vi "sonar222.vi"() -> ()   [LabVIEW 2020]
doc: "Use this template to build a producer/consumer design pattern. Use this template when you need to execute a process, such as data analysis, when a data source, such as a triggered acquisition, produces data at an uneven rate and you need to execute the process when the data becomes available."
uses:
  <vilib>/picture/picture.llb/imagedata.ctl
  <vilib>/MakerHub/LINX/Public/Utilities/Open Serial.vi
  <vilib>/MakerHub/LINX/Public/Sensors/Motion/Servo/Servo Open One Channel.vi
  <vilib>/MakerHub/LINX/Public/Sensors/Motion/Servo/Servo Set Pulse Width One Channel.vi
  <vilib>/MakerHub/LINX/Public/Sensors/Motion/Servo/Servo Close One Channel.vi
  <vilib>/MakerHub/LINX/LMH-LINX.lvlib
  <vilib>/MakerHub/LINX/Public/Sensors/Motion/Servo/Servo.lvlib
  <vilib>/MakerHub/LINX/Public/Sensors/Distance/Ultrasonic/Ultrasonic.lvlib
panel:
  out "2D picture":picture
  in  "STOP":bool
  out "Distance":dbl
  in  "Echo Pin":u8
  in  "Trig Pin":u8
  in  "Servo Pin":i32=10
  out "Angle":dbl
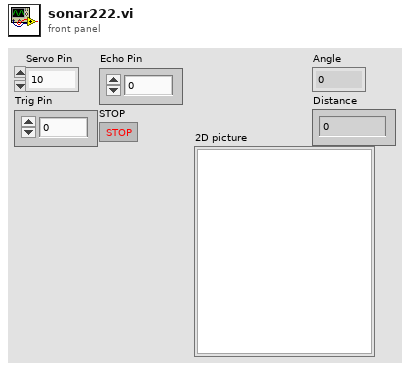
[diagram p1: front panel]
types:
  T1 = typedef "imagedata.ctl" = cluster{"image type":i32, "image depth":i32, "image":u8[], "mask":u8[], "colors":u32[], "Rectangle":cluster{"left":i16, "top":i16, "right":i16, "bottom":i16}}
  T2 = typedef "LMH-LINX.lvlib/LINX Ref.ctl" = cluster{"IO":T3, "Interface":T4, "LINX Device Config":T5}
  T3 = typedef "LMH-LINX.lvlib/Platform.ctl" = enum16{"Remote", "Local"}
  T4 = typedef "LMH-LINX.lvlib/Interface.ctl" = enum16{"Serial", "TCP"}
  T5 = typedef "LMH-LINX.lvlib/Device.lvlib/LINX Device Config.ctl" = cluster{"Interface":T4, "COM Port":refnum<visa-resource-name>, "TCP Configuration":T6, "Device Family":u8, "Device ID":u8, "Device Name":string, "TCP Ref":refnum<k5>, "Channels":T7}
  T6 = typedef "LMH-LINX.lvlib/Device.lvlib/TCP Config.ctl" = cluster{"IP Address":string, "Port":u16}
  T7 = typedef "LMH-LINX.lvlib/Channels.ctl" = cluster{"DI":u8[], "DO":u8[], "AI":u8[], "AO":u8[], "PWM":u8[], "QE":u8[], "UART":u8[], "I2C 2":u8[], "SPI":u8[], "CAN":u8[], "Servo":u8[], "AI Ref (V)":dbl, "AI Resolution (Bits)":u8, "AO Ref (V)":dbl, "AO Resolution (Bits)":u8}
  T8 = cluster{"maximum":dbl, "minimum":dbl, "clip to min":bool, "log?(F)":bool, "grid color":u32, "plot color":u32, "format and precision":cluster{"format":enum8{"Decimal", "Scientific", "Engineering", "Binary", "Octal", "Hex"}, "precision":u8}, "visible section":u16}
  T9 = typedef "LVBoundsTypeDef.ctl" = cluster{"Width":u32, "Height":u32}
  T10 = cluster{"pixel center":cluster{"x":i16, "y":i16}, "scale factors":cluster{"a":dbl, "b":dbl, "log?":bool}, "grid color":u32, "start angle":dbl, "end angle":dbl, "tick length":i16, "pixel radius":i32}
  T11 = cluster{"Distance (cm)":dbl, "Angle (deg)":dbl}[]
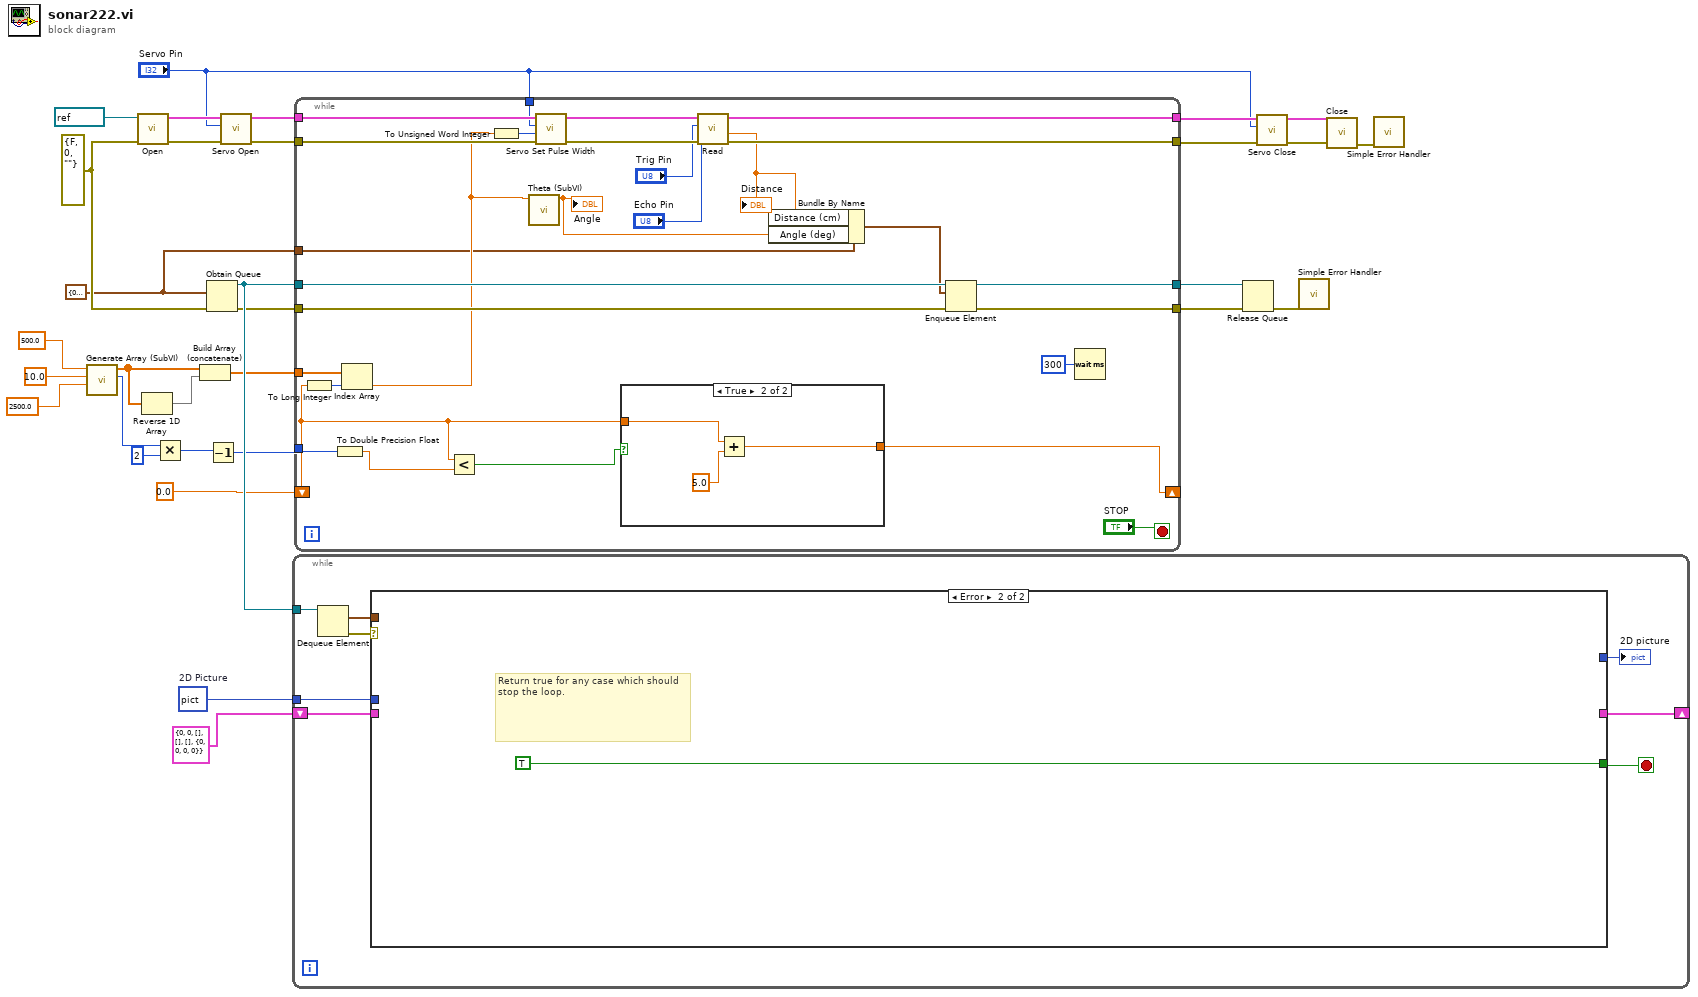
[diagram p0: block diagram]
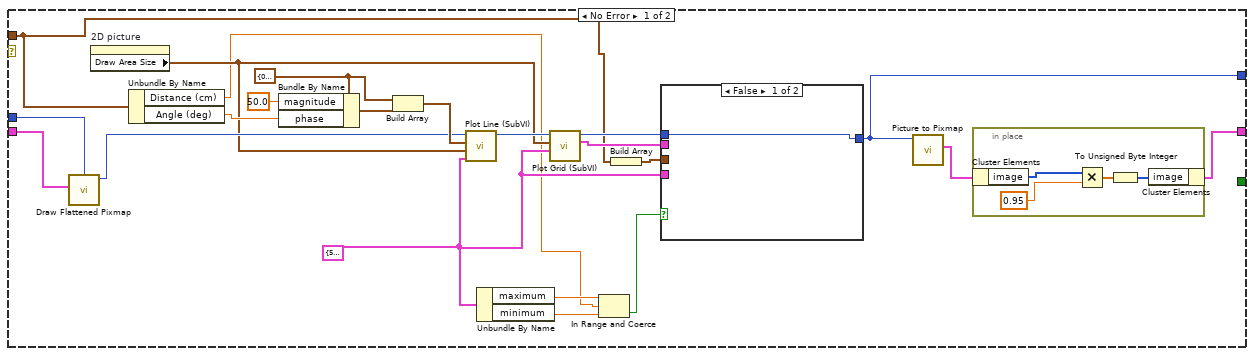
[diagram p2: hidden frame]
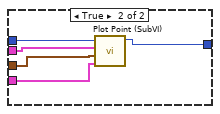
[diagram p3: hidden frame]
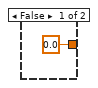
[diagram p4: hidden frame]
diagram:
  w1 = picture data[5B]  # 2D Picture
  w3 = cluster{"Distance (cm)":dbl, "Angle (deg)":dbl} {"Distance (cm)"=0.0, "Angle (deg)"=0.0}
  w17 = errorcluster {"status"=FALSE, "code"=0, "source"=""} ("Error Cluster In")
  n1 = call "Generate Array (SubVI).vi"("Final"=2500.0, "Step"=10.0, "Initial"=500.0) -> ("Array size"=w7:i32, "Array out"=w10:dbl[])  [unwired: 6 in, 1 out]
  n2 = call-poly <vilib>:"Open.vi"("Error In"=w17, "Serial Port"=refnum<visa-resource-name> "N/A") -> ("Error Out"=w23:errorcluster, "LINX Resource"=w27:T2)  [unwired: 7 in, 1 out]
  n3 = Reverse 1D Array(array=w10) -> (reversed array=w11:dbl[])
  n4 = Multiply(x=w7, y=2) -> (x*y=w5:i32)
  n5 = Build Array (concatenate)(w10, w11) -> (w9:dbl[])
  n6 = Obtain Queue(element data type=w3, error in (no error)=w17) -> (queue out=w31:refnum<queue>, error out=w30:errorcluster)  [unwired: 3 in, 1 out]
  n7 = Decrement(x=w5) -> (x-1=w4:i32)
  n8 = call-poly <vilib>:"Servo Open.vi"("Error In"=w23, "Servo Channel"="Servo Pin", "LINX Resource"=w27) -> ("Error Out"=w22:errorcluster, "LINX Resource"=w26:T2)  [unwired: 7 in]
  n9 = while {
    tunnel: w31 -> [w39]
    tunnel: w1 -> [w35]
    shift-right: [w33] -> _
    shift-left: T1 {"image type"=0, "image depth"=0, "image"=[], "mask"=[], "colors"=[], "Rectangle"={"left"=0, "top"=0, "right"=0, "bottom"=0}} -> [w36]
    stop <- w34 stop-if-true
    n10 = Dequeue Element(queue=w39) -> (element=w37:cluster{"Distance (cm)":dbl, "Angle (deg)":dbl}, error out=w38:errorcluster)  [unwired: 2 in, 2 out]
    n11 = case shown="Error" w38 {
      tunnel: w37 -> [w48 _]
      tunnel: [_ TRUE] -> w34
      tunnel: w36 -> [w61 _]
      tunnel: w35 -> [w55 _]
      tunnel: [w46 _] -> w33
      tunnel: [w45 _] -> w32
      frame No Error {
        w44 = T8 {"maximum"=50.0, "minimum"=0.0, "clip to min"=TRUE, "log?(F)"=FALSE, "grid color"=9868950, "plot color"=65280, "format and precision"={"format"=enum."Decimal", "precision"=0}, "visible section"=4} ("Polar Graph Attributes")
        w58 = cluster{"magnitude":dbl, "phase":dbl} {"magnitude"=0.0, "phase"=0.0}
        n12 = call <vilib>:"Draw Flattened Pixmap.vi"("image data"=w61, "picture"=w55) -> ("new picture"=w54:picture)  [unwired: 7 in]
        n13 = property on="2D picture" class="Pict"() -> ("Draw Area Size"=w52:T9)  [unwired: 2 in, 2 out]
        n14 = Unbundle By Name(w48) -> ("Distance (cm)"=w41:dbl, "Angle (deg)"=w60:dbl)
        n15 = Bundle By Name(cluster=w58, "magnitude"=50.0, "phase"=w60) -> (w57:cluster{"magnitude":dbl, "phase":dbl})
        n16 = Build Array(w58, w57) -> (w56:cluster{"magnitude":dbl, "phase":dbl}[])
        n17 = call "Plot Line (SubVI).vi"("Polar Graph Attributes"=w44, "Draw Area Size"=w52, "Polar Array"=w56, "new picture in"=w54) -> ("new picture out"=w53:picture)  [unwired: 7 in]
        n18 = Unbundle By Name(w44) -> ("maximum"=w43:dbl, "minimum"=w42:dbl)
        n19 = call "Plot Grid (SubVI).vi"("Polar Graph Attributes"=w44, "Draw Area Size"=w52, "new picture in"=w53) -> ("grid measurements"=w50:T10, "new picture out"=w51:picture)  [unwired: 7 in]
        n20 = In Range and Coerce(upper limit=w43, x=w41, lower limit=w42) -> (In Range?=w40:bool)  [unwired: 1 out]
        n21 = Build Array(w48) -> (w49:T11)
        n22 = case shown="False" w40 {
          tunnel: w51 -> [w66 w71]
          tunnel: w50 -> [_ w70]
          tunnel: w49 -> [_ w69]
          tunnel: w44 -> [_ w68]
          tunnel: [w66 w67] -> w45
          frame False {
          }
          frame True {
            n23 = call "Plot Point (SubVI).vi"("Polar Graph Attributes"=w68, "Array"=w69, "grid measurements"=w70, "new picture in"=w71) -> ("new picture"=w67:picture)  [unwired: 7 in]
          }
        }
        n24 = call <vilib>:"Picture to Pixmap.vi"("picture"=w45) -> ("image data"=w47:T1)  [unwired: 9 in, 1 out]
        n25 = in-place {
          # "Ghosting Effect"
          n26 = in-place-cluster #1(w47) -> ("image"=w65:u8[])
          n27 = Multiply(x=w65, y=0.95) -> (x*y=w63:dbl[])
          n28 = To Unsigned Byte Integer(number=w63) -> (unsigned 8bit integer=w62:u8[])
          n29 = in-place-cluster #1("image"=w62) -> (w46:T1)
        }
      }
      frame Error {
        # "Return true for any case which should stop the loop."
      }
    }
    "2D picture" <- w32
  }
  n30 = while {
    tunnel: w26 -> [w100]
    tunnel: [w98] -> w25
    tunnel: w22 -> [w97]
    tunnel: [w95] -> w21
    tunnel: w31 -> [w94]
    tunnel: [w93] -> w29
    tunnel: w30 -> [w92]
    tunnel: [w91] -> w28
    tunnel: "Servo Pin" -> [w90]
    tunnel: w9 -> [w89]
    shift-right: [w74] -> _
    shift-left: 0.0 -> [w75]
    tunnel: w4 -> [w87]
    tunnel: w3 -> [w80]
    stop <- "STOP" stop-if-true
    n31 = To Long Integer(number=w75) -> (32bit integer=w88:i32)
    n32 = To Double Precision Float(number=w87) -> (double precision float=w76:dbl)
    n33 = Index Array(array=w89, index=w88) -> (element=w85:dbl)
    n34 = Less?(x=w75, y=w76) -> (x < y?=w77:bool)
    n35 = To Unsigned Word Integer(number=w85) -> (unsigned 16bit integer=w86:u16)
    n36 = call "Theta (SubVI).vi"("PWM"=w85) -> ("Theta"=w81:dbl)  [unwired: 9 in, 1 out]
    "Angle" <- w81
    n37 = call-poly <vilib>:"Servo Set Pulse Width.vi"("Error In"=w97, "Pulse Width (uS)"=w86, "Servo Channel"=w90, "LINX Resource"=w100) -> ("Error Out"=w96:errorcluster, "LINX Resource"=w99:T2)  [unwired: 6 in]
    n38 = case shown="True" w77 {
      tunnel: w75 -> [_ w103]
      tunnel: [0.0 w102] -> w74
      frame False {
      }
      frame True {
        n39 = Add(x=w103, y=5.0) -> (x+y=w102:dbl)
      }
    }
    n40 = call <vilib>:"Read.vi"("Error In"=w96, "DO Channel"="Echo Pin", "DI Channel"="Trig Pin", "LINX Resource"=w99) -> ("Error Out"=w95:errorcluster, "Centimeters"=w82:dbl, "LINX Resource"=w98:T2)  [unwired: 4 in, 1 out]
    "Distance" <- w82
    n41 = Bundle By Name(cluster=w80, "Distance (cm)"=w82, "Angle (deg)"=w81) -> (w79:cluster{"Distance (cm)":dbl, "Angle (deg)":dbl})
    n42 = Enqueue Element(queue=w94, element=w79, error in (no error)=w92) -> (queue out=w93:refnum<queue>, error out=w91:errorcluster)  [unwired: 1 in, 1 out]
    n43 = Wait (ms)(milliseconds to wait=u32 300) -> ()  [unwired: 1 out]
  }
  n44 = Release Queue(queue=w29, error in (no error)=w28) -> (error out=w16:errorcluster)  [unwired: 1 in, 2 out]
  n45 = call-poly <vilib>:"Servo Close.vi"("Error In"=w21, "Servo Channel"="Servo Pin", "LINX Resource"=w25) -> ("Error Out"=w20:errorcluster, "LINX Resource"=w24:T2)  [unwired: 7 in]
  n46 = call <vilib>:"Simple Error Handler.vi"("error in (no error)"=w16) -> ()  [unwired: 4 in, 5 out]
  n47 = call <vilib>:"Close.vi"("Error In"=w20, "LINX Resource"=w24) -> ("Error Out"=w19:errorcluster)  [unwired: 9 in]
  n48 = call <vilib>:"Simple Error Handler.vi"("error in (no error)"=w19) -> ()  [unwired: 4 in, 5 out]
